vi "修改密码.vi"(10 "旧密码in":string) -> (1 "取消":bool, 2 "新密码out":string)   [LabVIEW 2020]
panel:
  in  "确认密码":string
  in  "Btn_Exit":bool
  in  "Btn_Confirm":bool
  in  "新密码":string
  in  "旧密码":string
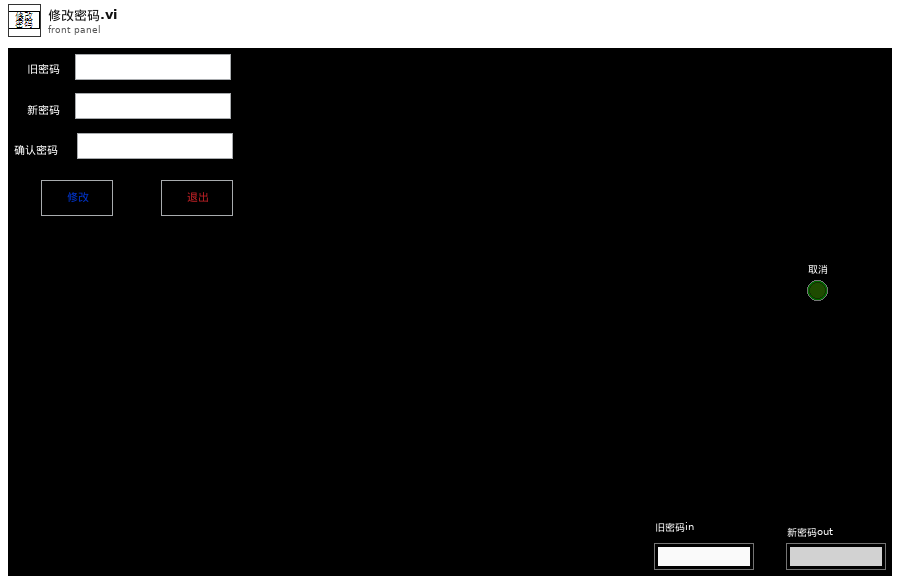
[diagram p1: front panel]
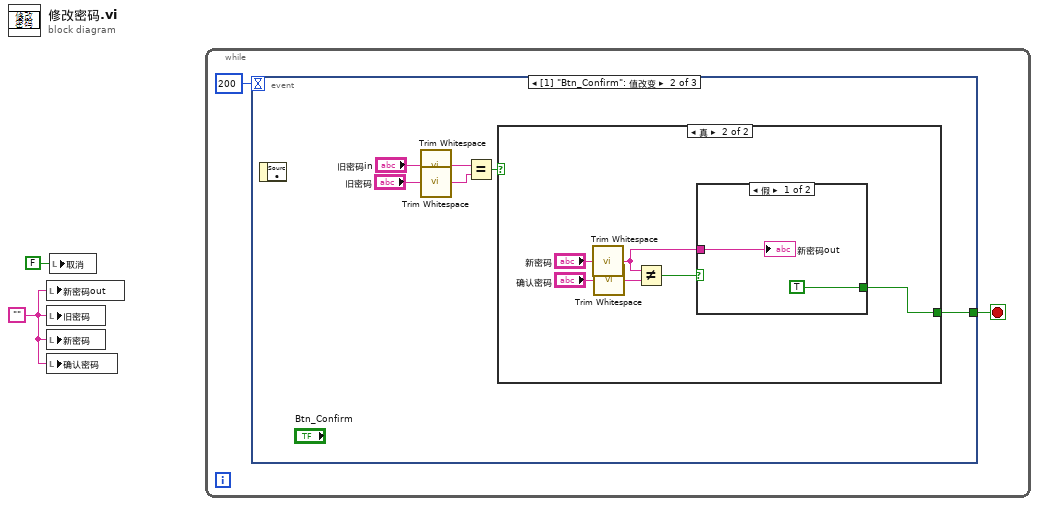
[diagram p0: block diagram]
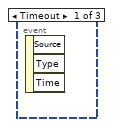
[diagram p2: hidden frame]
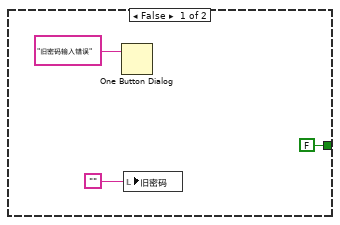
[diagram p3: hidden frame]
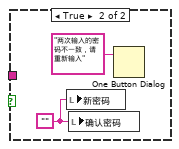
[diagram p4: hidden frame]
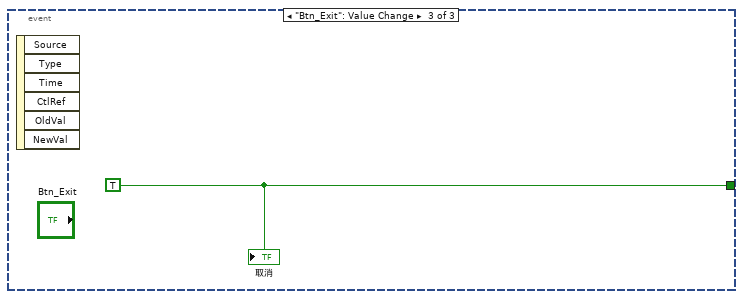
[diagram p5: hidden frame]
diagram:
  w1 = "" ("用户名")
  n1 = local write "新密码out"(w1) -> ()
  n2 = local write "旧密码"(w1) -> ()
  n3 = local write "新密码"(w1) -> ()
  n4 = local write "确认密码"(w1) -> ()
  n5 = local write "取消"(FALSE ("取消")) -> ()
  n6 = while {
    stop <- w3 stop-if-true
    n7 = event shown="[1] \"Btn_Confirm\": 值改变" {
      selector: _ -> [_ _ _]
      dyn-events: _ -> [_ _ _]
      timeout: 200 -> [_ _ _]
      tunnel: [_ w10 w24] -> w3
      event Timeout {
        n8 = event-data() -> ()  [unwired: 1 in, 3 out]
      }
      event "Btn_Confirm": Value Change {
        n9 = event-data() -> ()  [unwired: 1 in, 1 out]
        n10 = call <vilib>:"Trim Whitespace.vi"("string"="旧密码in") -> ("trimmed string"=w5:string)  [unwired: 1 in]
        n11 = call <vilib>:"Trim Whitespace.vi"("string"="旧密码") -> ("trimmed string"=w6:string)  [unwired: 1 in]
        n12 = Equal?(x=w5, y=w6) -> (x = y?=w7:bool)
        n13 = case shown="真" w7 {
          tunnel: [FALSE w17] -> w10
          frame False {
            n14 = One Button Dialog(message="旧密码输入错误" ("消息")) -> ()  [unwired: 1 in, 1 out]
            n15 = local write "旧密码"("" ("用户名")) -> ()
          }
          frame True {
            n16 = call <vilib>:"Trim Whitespace.vi"("string"="新密码") -> ("trimmed string"=w15:string)  [unwired: 1 in]
            n17 = call <vilib>:"Trim Whitespace.vi"("string"="确认密码") -> ("trimmed string"=w14:string)  [unwired: 1 in]
            n18 = Not Equal?(x=w15, y=w14) -> (x != y?=w18:bool)
            n19 = case shown="假" w18 {
              tunnel: [TRUE _] -> w17
              tunnel: w15 -> [w20 _]
              frame False {
                "新密码out" <- w20
              }
              frame True {
                w22 = ""
                n20 = local write "新密码"(w22) -> ()
                n21 = local write "确认密码"(w22) -> ()
                n22 = One Button Dialog(message="两次输入的密码不一致，请重新输入" ("消息")) -> ()  [unwired: 1 in, 1 out]
              }
            }
          }
        }
      }
      event "Btn_Exit": Value Change {
        w24 = TRUE ("取消")
        n23 = event-data() -> ()  [unwired: 1 in, 6 out]
        "取消" <- w24
      }
    }
  }
